vi "FileIO-Write Settings.vi"(0 "Parameters":T1, 1 "Setting Files":path, 7 "Prompt? (T)":bool=TRUE, 11 "error in (no error)":errorcluster) -> (4 "selected path":path, 8 "saved":bool, 15 "error out":errorcluster)   [LabVIEW 2015]
uses:
  Pathfinder/SNF/LV Source/Typedefs/SNF-Parameters.ctl
  Pathfinder/SNF/LV Source/Typedefs/SNF-Stimulus.ctl
  Pathfinder/SNF/LV Source/Typedefs/SNF-Mapping.ctl
  User Variables/User Variable.ctl
  Pathfinder/SNF/LV Source/Typedefs/SNF-Rules.ctl
  <vilib>/Utility/sysdir.llb/System Directory Type.ctl
panel:
  out "Version":i32
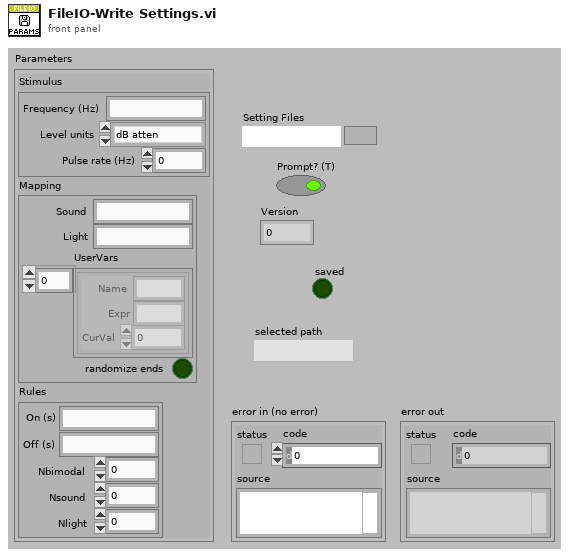
[diagram p1: front panel]
types:
  T1 = typedef "SNF-Parameters.ctl" = cluster{"Stimulus":T2, "Mapping":T3, "Rules":T5}
  T2 = typedef "SNF-Stimulus.ctl" = cluster{"Frequency (Hz)":string, "Level units":enum16{"dB atten", "dB SPL"}, "Pulse rate (Hz)":dbl}
  T3 = typedef "SNF-Mapping.ctl" = cluster{"Sound":string, "Light":string, "randomize ends":bool, "UserVars":T4[]}
  T4 = typedef "User Variable.ctl" = cluster{"Name":string, "Expr":string, "CurVal":dbl}
  T5 = typedef "SNF-Rules.ctl" = cluster{"On (s)":string, "Off (s)":string, "Nbimodal":i32, "Nsound":i32, "Nlight":i32}
  T6 = typedef "System Directory Type.ctl" = i32
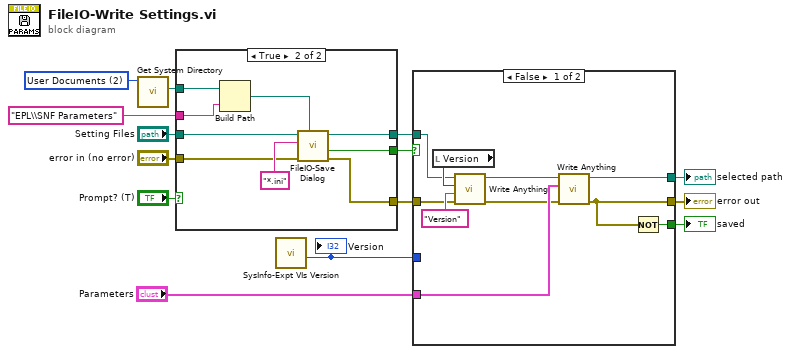
[diagram p0: block diagram]
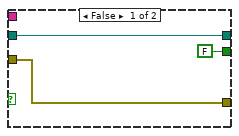
[diagram p2: hidden frame]
diagram:
  w3 = T6 2 items=["User Home"=0, "User Desktop"=1, "User Documents"=2, "User Application Data"=3, "User Preferences"=4, "User Temporary"=5, "Public Documents"=6, "Public Application Data"=7, "Public Preferences"=8, "Public Cache"=13, "System Core Libraries"=9, "System Installed Libraries"=10, "Application Files"=11, "Boot Volume Root"=12] ("system directory type")
  n1 = call <vilib>:"Get System Directory.vi"("system directory type"=w3) -> ("system directory"=w2:path)  [unwired: 10 in]
  n2 = case shown="True" "Prompt? (T)" {
    tunnel: [FALSE ("cancelled") w26] -> w12
    tunnel: [w16 w25] -> w11
    tunnel: [w15 w24] -> w8
    tunnel: "Setting Files" -> [w16 w22]
    tunnel: "error in (no error)" -> [w15 w21]
    tunnel: w2 -> [_ w20]
    tunnel: "EPL\\SNF Parameters" ("name or relative path") -> [_ w19]
    frame False {
    }
    frame True {
      n3 = Build Path(base path=w20, name or relative path=w19) -> (appended path=w18:path)
      n4 = call "FileIO-Save Dialog.vi"("Default Folder"=w18, "error in"=w21, "pattern (all files)"="*.ini", "Start path"=w22) -> ("error out"=w24:errorcluster, "cancelled"=w26:bool, "selected path"=w25:path)  [unwired: 5 in]
    }
  }
  n5 = call "SysInfo-Expt VIs Version.vi"() -> ("Expt VIs Version out"=w7:i32)  [unwired: 11 in]
  "Version" <- w7
  n6 = case shown="False" w12 {
    tunnel: [w27 w38] -> w14
    tunnel: "Parameters" -> [w36 _]
    tunnel: w11 -> [w33 w37]
    tunnel: w8 -> [w32 w38]
    tunnel: w7 -> [_ _]
    tunnel: [w31 _] -> w6
    tunnel: [w28 w37] -> w5
    frame False {
      n7 = local read "Version"() -> (w35:i32)
      n8 = call "Write Anything.vi"("Error In"=w32, "Section Name (Name of \"Anything\")"="Version" ("Section Name (Name of \"Anything\")"), "Anything"=w35, "Path (dialog)"=w33) -> ("Error Out"=w30:errorcluster, "Path out"=w29:path)  [unwired: 6 in]
      n9 = call "Write Anything.vi"("Error In"=w30, "Anything"=w36, "Path (dialog)"=w29) -> ("Error Out"=w27:errorcluster, "Path out"=w28:path)  [unwired: 7 in]
      n10 = Not(x=w27) -> (.not. x?=w31:bool)
    }
    frame True {
    }
  }
  "error out" <- w14
  "saved" <- w6
  "selected path" <- w5
